vi "Find Stop Module.vi"(8 "error in":errorcluster, 11 "Event vi Ref":refnum<vi>) -> (0 "error out":errorcluster, 2 "Cloneable?":bool, 3 "Stop Module":path)   [LabVIEW 2020, in "DQMH_API.lvlib"]
uses:
  DQMH_API.lvlib
  <vilib>/Utility/error.llb/Error Cluster From Error Code.vi
  <vilib>/ErrorRing/Error Ring.xnode
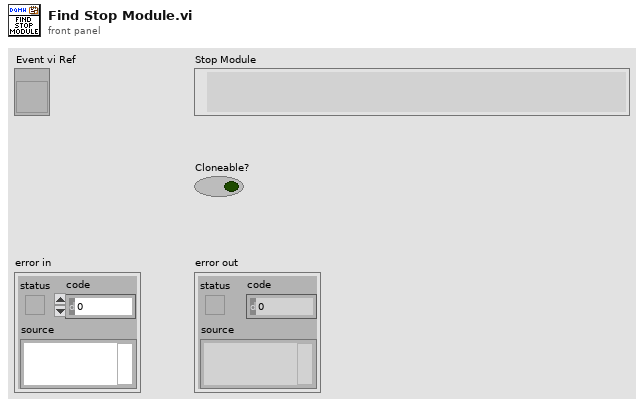
[diagram p1: front panel]
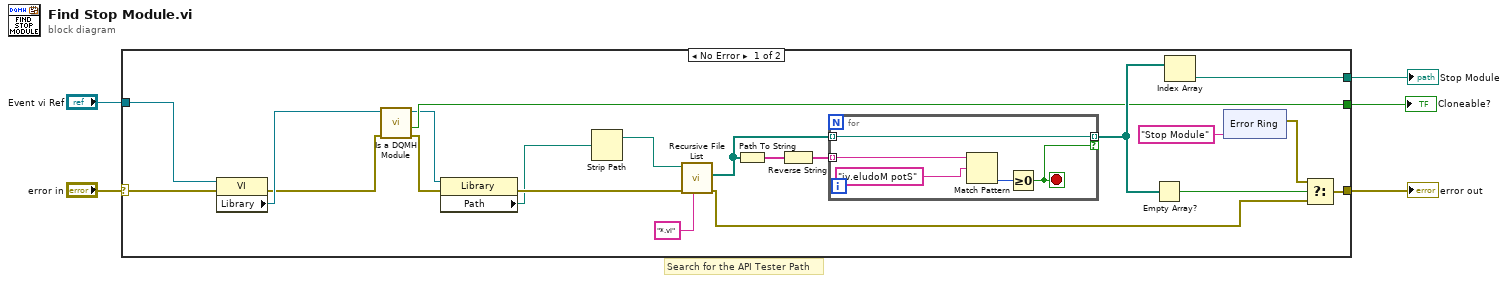
[diagram p0: block diagram]
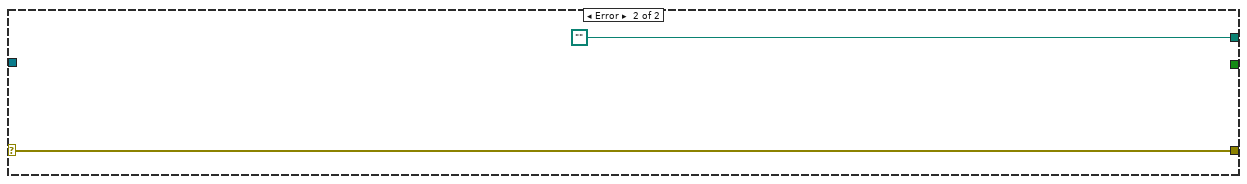
[diagram p2: hidden frame]
diagram:
  # "Search for the API Tester Path"
  n1 = case shown="No Error" "error in" {
    selector: "error in" -> [w23 w40]
    tunnel: [w17 path ""] -> w3
    tunnel: [w24 w40] -> w4
    tunnel: "Event vi Ref" -> [w12 _]
    tunnel: [w7 _] -> w1
    frame No Error {
      n2 = property class="VI"(reference=w12, error in=w23) -> (error out=w9:errorcluster, "Library"=w10:refnum<vi>)  [unwired: 1 out]
      n3 = call "Is a DQMH Module.vi"("error in"=w9, "Library"=w10) -> ("error out"=w8:errorcluster, "Cloneable?"=w7:bool, "Library Refnum"=w6:refnum<vi>)  [unwired: 6 in, 1 out]
      n4 = property class="Library"(reference=w6, error in=w8) -> (error out=w22:errorcluster, "Path"=w13:path)  [unwired: 1 out]
      n5 = Strip Path(path=w13) -> (stripped path=w14:path)  [unwired: 1 out]
      n6 = call <vilib>:"Recursive File List.vi"("pattern"="*.vi", "error in (no error)"=w22, "Folder Path"=w14) -> ("error out"=w25:errorcluster, "All Files in Dir"=w18:path[])  [unwired: 4 in, 3 out]
      n7 = Path To String(path=w18) -> (string=w20:string[])
      n8 = Reverse String(1:w20) -> (0:w19:string[])
      n9 = for {
        tunnel: w19 -> [w36] mode=indexing
        tunnel: w18 -> [w38] mode=indexing
        tunnel: [w38] -> w16 mode=indexing if=w34
        stop <- w34 stop-if-true
        n10 = Match Pattern(string=w36, regular expression="iv.eludoM potS") -> (offset past match=w35:i32)  [unwired: 1 in, 3 out]
        n11 = Greater Or Equal To 0?(x=w35) -> (x >= 0?=w34:bool)
      }
      n12 = Empty Array?(array=w16) -> (empty?=w15:bool)
      n13 = Index Array(array=w16) -> (element=w17:path)  [unwired: 1 in]
      n14 = xnode "Error Ring"("parameter 0"="Stop Module") -> ("error out"=w26:errorcluster)
      n15 = Select(t=w26, s=w15, f=w25) -> (s? t:f=w24:errorcluster)
    }
    frame Error {
    }
  }
  "Stop Module" <- w3
  "error out" <- w4
  "Cloneable?" <- w1
